vi "crio_FPGA_HX711_DMA.vi"() -> ()   [LabVIEW 2019]
uses:
  hx711/Data.ctl
  hx711/State.ctl
  <vilib>/rvi/Emulation/niFpgaSctlEmulationGetInTimedLoop.vi
  <vilib>/rvi/Emulation/niFpgaProcessEmulError.vi
  <vilib>/rvi/eio/common/nirviEmuTemplateMethod_errors.vi
  <vilib>/rvi/Emulation/niFpgaGetClockAttributes.vi
  <vilib>/rvi/Emulation/niFpgaEmulationReportErrorSimple.vi
  <vilib>/rvi/Emulation/niFpgaCriticalErrorInLSC.vi
  <vilib>/rvi/interface/RandomDataEmulation/niFpgaRandomDataHandleErrors.vi
  <vilib>/eio/EIOMethodNode/EIOMethodNode.xnode
  <vilib>/eio/EIONode/EIONode.xnode
  <vilib>/rvi/DataTransferAndStorage/Container/XNode/niFpgaContainer.xnode
  <vilib>/rvi/interface/RandomDataEmulation/nirviRandomDataFpgaReadWriteTemplate.vi
panel:
  out "Data array":i32[](array[numeric])
  in  "PowerDown?":bool
  out "Data":i32
  in  "Gain/ChannelSelect":T1(ring)
  in  "stop":bool
  # "1000, fully retract\n2000, fully extend\nbetween, inner PD control"
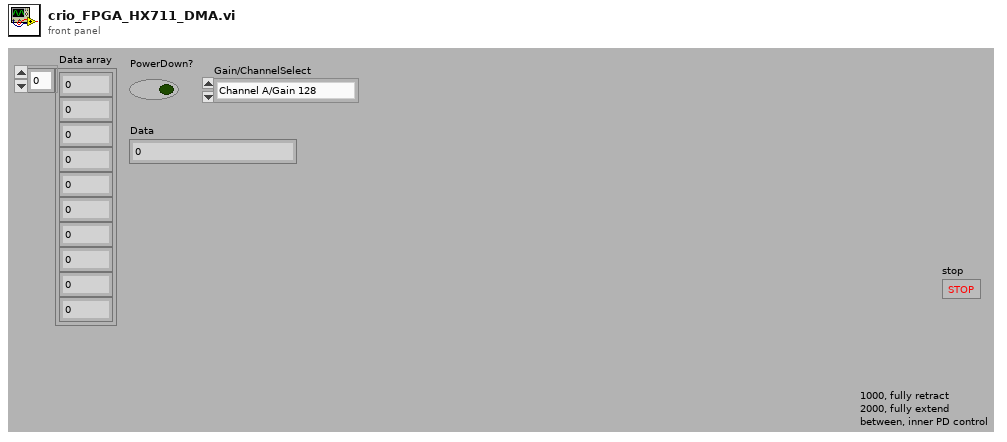
[diagram p1: front panel]
types:
  T1 = enum16{"Channel A/Gain 128", "Channel A/Gain 64", "Channel B/Gain 32"}
  T2 = typedef "State.ctl" = enum16{"PowerUp", "PowerDown", "Gain/ChannelSelect", "ReadData", "ClockLow", "ClockHigh", "ConvertData", "RetrievalReady?"}
  T3 = typedef "Data.ctl" = cluster{"DT":bool, "SCK":bool, "2's Data":i32, "PulseCount":u8, "DelayTime":u8, "Data":i32, "PowerDown?":bool, "Gain/ChannelSelect":enum16{"Channel A/Gain 128", "Channel A/Gain 64", "Channel B/Gain 32"}}
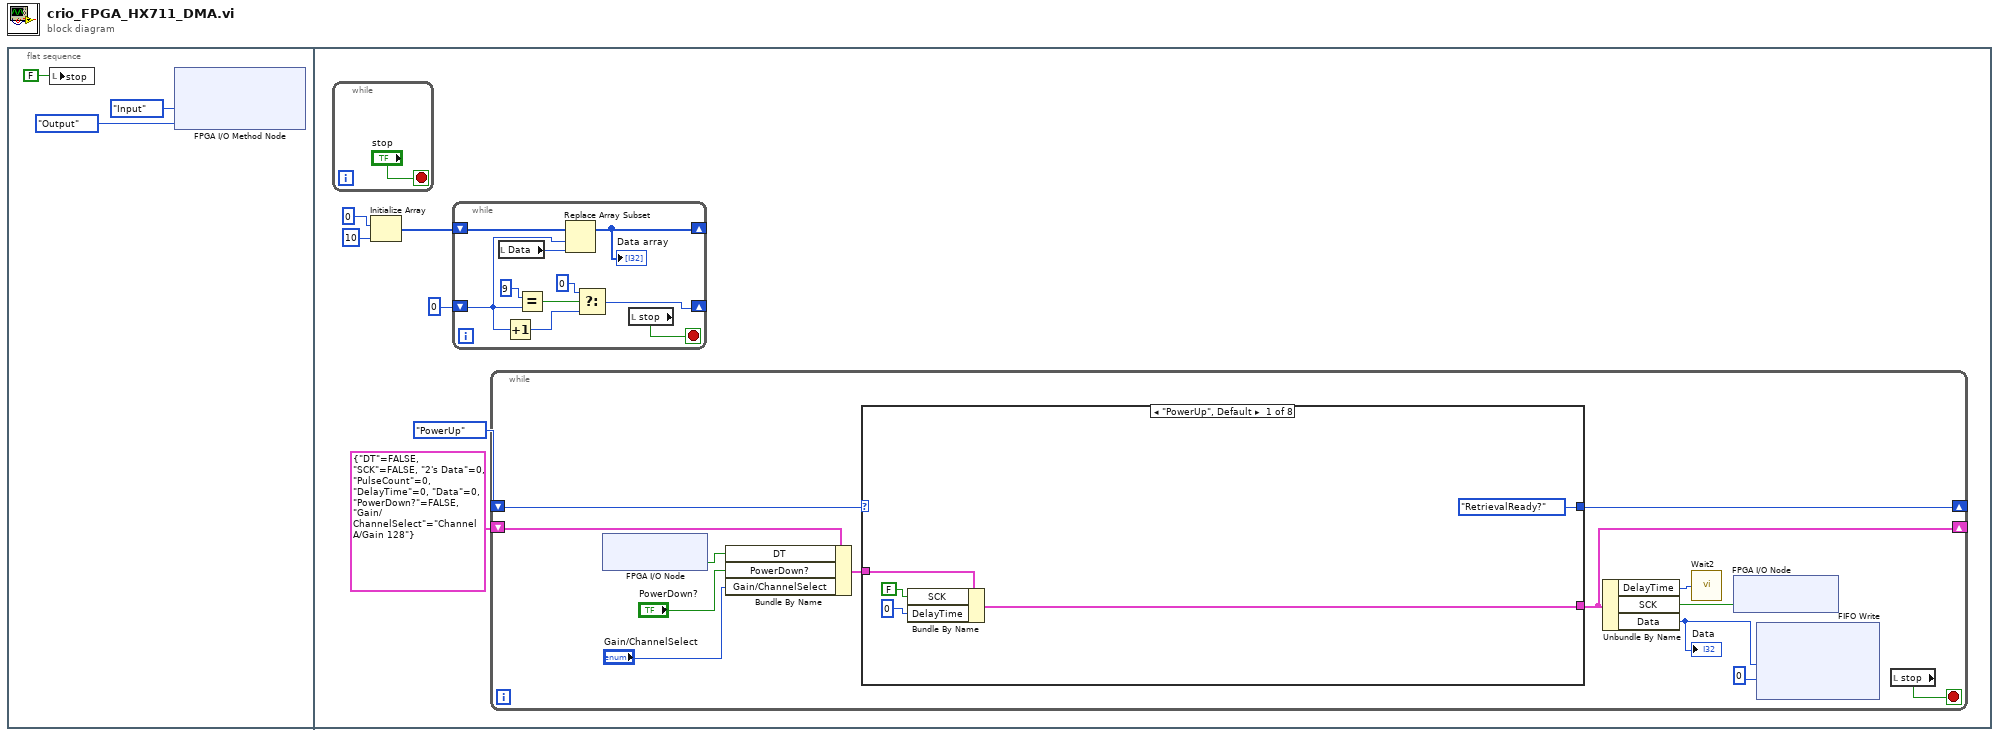
[diagram p0: block diagram]
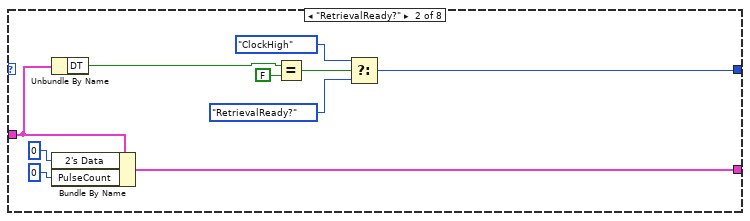
[diagram p2: hidden frame]
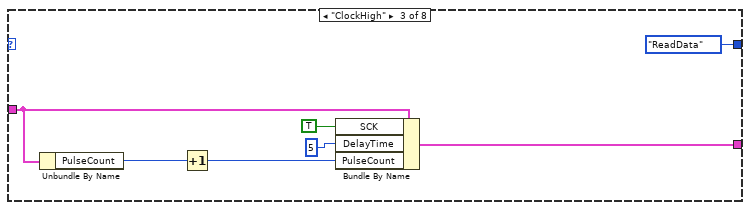
[diagram p3: hidden frame]
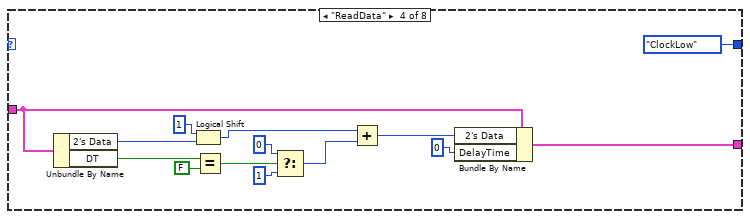
[diagram p4: hidden frame]
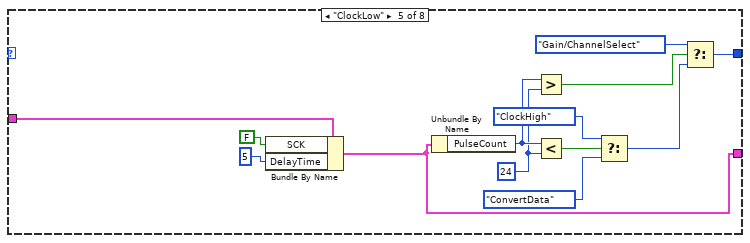
[diagram p5: hidden frame]
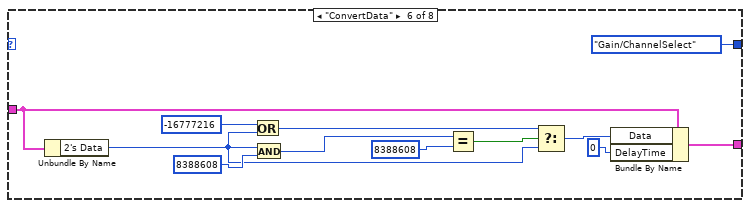
[diagram p6: hidden frame]
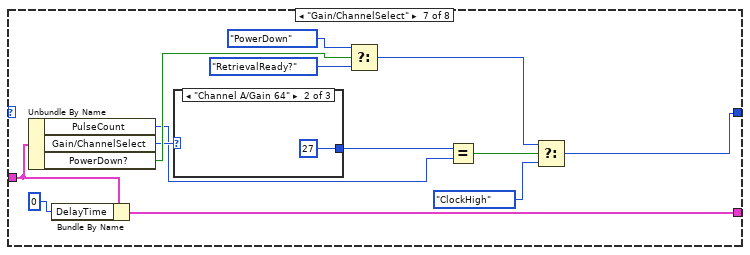
[diagram p7: hidden frame]
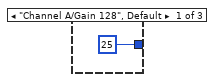
[diagram p8: hidden frame]
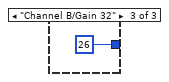
[diagram p9: hidden frame]
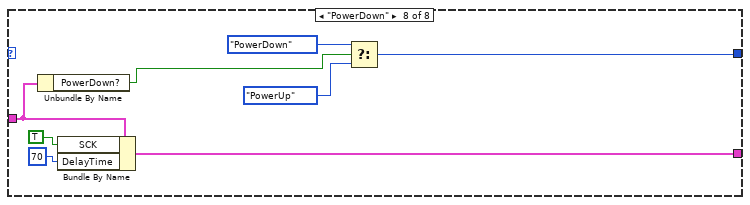
[diagram p10: hidden frame]
diagram:
  n1 = flat-sequence {
    frame #0 {
      n2 = local write "stop"(FALSE ("stop")) -> ()
      n3 = xnode "FPGA I/O Method Node"("DIO 7:4"=enum8{"No Change", "Input", "Output"}."Input", "DIO 3:0"=enum8{"No Change", "Input", "Output"}."Output") -> ()  [unwired: 1 in, 1 out]
    }
    frame #1 {
      n4 = while {
        stop <- "stop" stop-if-true
      }
      n5 = Initialize Array(0 ("Data"), 10 ("dimension size")) -> (w9:i32[])
      n6 = while {
        shift-right: [w12] -> _
        shift-left: w9 -> [w13]
        shift-right: [w18] -> _
        shift-left: 0 ("index") -> [w14]
        stop <- w11 stop-if-true
        n7 = local read "Data"() -> (w20:i32)
        n8 = Increment(x=w14) -> (x+1=w17:i32)
        n9 = Equal?(x=9, y=w14) -> (x = y?=w15:bool)
        n10 = Replace Array Subset(array=w13, new element=w20, index=w14) -> (w12:i32[])
        "Data array" <- w12
        n11 = Select(t=0 ("index"), s=w15, f=w17) -> (s? t:f=w18:i32)
        n12 = local read "stop"() -> (w11:bool)
      }
      n13 = while {
        shift-right: [w25] -> _
        shift-left: T3 {"DT"=FALSE, "SCK"=FALSE, "2's Data"=0, "PulseCount"=0, "DelayTime"=0, "Data"=0, "PowerDown?"=FALSE, "Gain/ChannelSelect"=enum."Channel A/Gain 128"} ("Data") -> [w30]
        shift-right: [w31] -> _
        shift-left: State."PowerUp" ("State") -> [w33]
        stop <- w23 stop-if-true
        n14 = xnode "FPGA I/O Node"() -> ("Mod8/DIO0"=w28:bool)  [unwired: 1 in, 1 out]
        n15 = Bundle By Name(cluster=w30, "DT"=w28, "PowerDown?"="PowerDown?", "Gain/ChannelSelect"="Gain/ChannelSelect") -> (w29:T3)
        n16 = case shown="\"PowerUp\", Default" w33 {
          tunnel: w29 -> [w38 w42 w51 w56 w82 w87 w97 w112]
          tunnel: [w36 w41 w55 w58 w77 w86 w96 w118] -> w25
          tunnel: [State."RetrievalReady?" ("State") w44 State."ReadData" ("State") State."ClockLow" ("State") w78 State."Gain/ChannelSelect" ("State") w104 w113] -> w31
          frame "PowerUp", Default {
            n17 = Bundle By Name(cluster=w38, "SCK"=FALSE, "DelayTime"=u8 0) -> (w36:T3)
          }
          frame "RetrievalReady?" {
            n18 = Unbundle By Name(w42) -> ("DT"=w48:bool)
            n19 = Bundle By Name(cluster=w42, "2's Data"=0, "PulseCount"=u8 0) -> (w41:T3)
            n20 = Equal?(x=w48, y=FALSE) -> (x = y?=w43:bool)
            n21 = Select(t=State."ClockHigh" ("State"), s=w43, f=State."RetrievalReady?" ("State")) -> (s? t:f=w44:T2)
          }
          frame "ClockHigh" {
            n22 = Unbundle By Name(w51) -> ("PulseCount"=w50:u8)
            n23 = Increment(x=w50) -> (x+1=w49:u8)
            n24 = Bundle By Name(cluster=w51, "SCK"=TRUE, "DelayTime"=u8 5, "PulseCount"=w49) -> (w55:T3)
          }
          frame "ReadData" {
            n25 = Unbundle By Name(w56) -> ("2's Data"=w69:i32, "DT"=w67:bool)
            n26 = Logical Shift(y=i16 1, x=w69) -> (x << y=w64:i32)
            n27 = Equal?(x=w67, y=FALSE ("SCK")) -> (x = y?=w65:bool)
            n28 = Select(t=0 ("DelayTime"), s=w65, f=1 ("DelayTime")) -> (s? t:f=w61:i32)
            n29 = Add(x=w64, y=w61) -> (x+y=w60:i32)
            n30 = Bundle By Name(cluster=w56, "2's Data"=w60, "DelayTime"=u8 0) -> (w58:T3)
          }
          frame "ClockLow" {
            w71 = u8 24 ("y")
            n31 = Bundle By Name(cluster=w82, "SCK"=FALSE, "DelayTime"=u8 5) -> (w77:T3)
            n32 = Unbundle By Name(w77) -> ("PulseCount"=w72:u8)
            n33 = Greater?(x=w72, y=w71) -> (0:w70:bool)
            n34 = Less?(x=w72, y=w71) -> (x < y?=w74:bool)
            n35 = Select(t=State."ClockHigh" ("State"), s=w74, f=State."ConvertData" ("State")) -> (s? t:f=w73:T2)
            n36 = Select(t=State."Gain/ChannelSelect" ("State"), s=w70, f=w73) -> (s? t:f=w78:T2)
          }
          frame "ConvertData" {
            n37 = Unbundle By Name(w87) -> ("2's Data"=w88:i32)
            n38 = Or(x=-16777216 ("y"), y=w88) -> (x .or. y?=w89:i32)
            n39 = And(x=w88, y=8388608) -> (x .and. y?=w93:i32)
            n40 = Equal?(x=w93, y=8388608) -> (x = y?=w91:bool)
            n41 = Select(t=w89, s=w91, f=w88) -> (s? t:f=w84:i32)
            n42 = Bundle By Name(cluster=w87, "Data"=w84, "DelayTime"=u8 0) -> (w86:T3)
          }
          frame "Gain/ChannelSelect" {
            n43 = Unbundle By Name(w97) -> ("PulseCount"=w100:u8, "Gain/ChannelSelect"=w102:T1, "PowerDown?"=w103:bool)
            n44 = Bundle By Name(cluster=w97, "DelayTime"=u8 0) -> (w96:T3)
            n45 = case shown="\"Channel A/Gain 64\"" w102 {
              tunnel: [u8 25 ("PulseCount") u8 27 ("PulseCount") u8 26 ("PulseCount")] -> w101
              frame "Channel A/Gain 128", Default {
              }
              frame "Channel A/Gain 64" {
              }
              frame "Channel B/Gain 32" {
              }
            }
            n46 = Select(t=State."PowerDown" ("State"), s=w103, f=State."RetrievalReady?" ("State")) -> (s? t:f=w99:T2)
            n47 = Equal?(x=w101, y=w100) -> (x = y?=w98:bool)
            n48 = Select(t=w99, s=w98, f=State."ClockHigh" ("State")) -> (s? t:f=w104:T2)
          }
          frame "PowerDown" {
            n49 = Unbundle By Name(w112) -> ("PowerDown?"=w111:bool)
            n50 = Bundle By Name(cluster=w112, "SCK"=TRUE, "DelayTime"=u8 70) -> (w118:T3)
            n51 = Select(t=State."PowerDown" ("State"), s=w111, f=State."PowerUp" ("State")) -> (s? t:f=w113:T2)
          }
        }
        n52 = Unbundle By Name(w25) -> ("DelayTime"=w32:u8, "SCK"=w24:bool, "Data"=w21:i32)
        "Data" <- w21
        n53 = call "Wait2"("Count(uSec)"=w32) -> ()  [unwired: 1 out]
        n54 = xnode "FPGA I/O Node"("Mod8/DIO1"=w24) -> ()  [unwired: 1 in, 1 out]
        n55 = xnode ("FIFO Write")("Element"=w21, "Timeout"=0) -> ()  [unwired: 1 in, 2 out]
        n56 = local read "stop"() -> (w23:bool)
      }
    }
  }
